vi "GetStopCode.vi"(8 "error in":errorcluster, 11 "VISA resource name":refnum<visa-resource-name>) -> (0 "error out":errorcluster, 1 "Stop code":i32, 2 "Stop code":string, 3 "VISA resource name out":refnum<visa-resource-name>)   [LabVIEW 2023, in "Thermotron 8800.lvlib"]
doc: "SCOD\nCommand name: Send stop code\nCommand type: System status\nDescription: The stop code identifies the cause of the most recent transition to the stop state. The stop codes are defined as follows:\n0 Cold boot power up. The 8800 memory has been initialized.\n1 Currently running. Not in stop. \n2 Stop key pressed. \n3 End of test. \n4 External input. An input defined as stop has been activated. \n5 Computer interface. The 8800 received the stop command. \n6 Open input. A thermocouple or analog input is open. \n7 Process alarm. A process alarm setting has been exceeded. \n8 System Monitor trip. \n9 Power fail recovery. The selected power fail recover mode was stop. \n10 Therm-Alarm trip.\nSyntax: SCOD?\nData type: Integer\nQuery example: SCOD?\n8800 response: 3 (The currently loaded test has ended.)"
uses:
  Thermotron 8800.lvlib
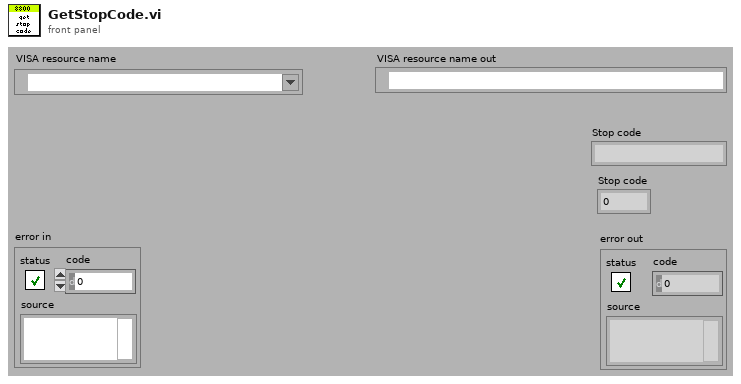
[diagram p1: front panel]
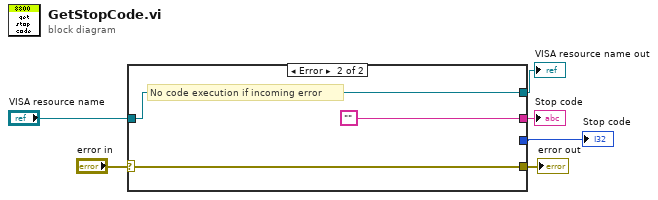
[diagram p0: block diagram]
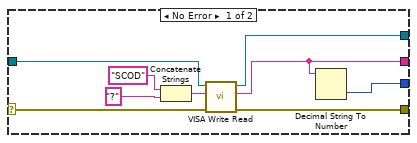
[diagram p2: hidden frame]
diagram:
  n1 = case shown="Error" "error in" {
    selector: "error in" -> [w13 w18]
    tunnel: [w12 w18] -> w5
    tunnel: "VISA resource name" -> [w11 w16]
    tunnel: [w10 w16] -> w3
    tunnel: [w8 ""] -> w2
    tunnel: [w7 _] -> w1
    frame No Error {
      n2 = Concatenate Strings("SCOD" ("8800 Command"), "?" ("8800 Command")) -> (w15:string)
      n3 = call "VISA Write Read.vi"("error in (no error)"=w13, "8800 Command"=w15, "VISA Refnum in"=w11) -> ("error out"=w12:errorcluster, "read buffer"=w8:string, "VISA Refnum out"=w10:refnum<visa-resource-name>)  [unwired: 6 in]
      n4 = Decimal String To Number(string=w8) -> (number=w7:i32)  [unwired: 2 in, 1 out]
    }
    frame Error {
      # "No code execution if incoming error"
    }
  }
  "error out" <- w5
  "VISA resource name out" <- w3
  "Stop code" <- w2
  "Stop code" <- w1
